vi "DoorProc_02.vi"(8 "error in":errorcluster, 11 "Cluster":T1) -> (0 "error out":errorcluster, 2 "Card Info":string, 3 "Certificate":bool=TRUE)   [LabVIEW 2011]
uses:
  Enumerator/CmdType.ctl
  DLL/Certificate_01.vi
  Interface/SockeHook/Hook_01.vi
  Variable/gSIM.vi
  Interface/SockeHook/Hook_02.vi
  Look-up/CardInfo/SPR_02.vi
  DLL/Certificate_02.vi
  Variable/gSEL.vi
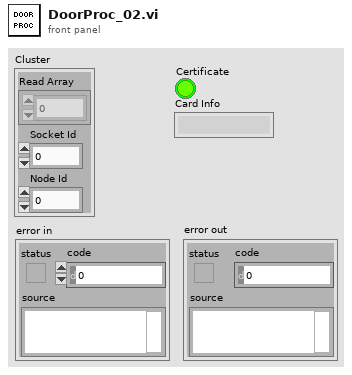
[diagram p1: front panel]
types:
  T1 = cluster{"Read Array":u8[], "Socket Id":u8, "Node Id":u8}
  T2 = enum16{"Open", "Verify", "Password", "Log", "Close"}
  T3 = enum16{"Open", "R", "W", "R->W", "W->R", "Close"}
  T4 = typedef "CmdType.ctl" = enum16{"GetEventLog", "DelTransaction", "InvalidMessage", "RelayControl", "RelayOff", "RelayOn", "VaildMessage", "EventPolling", "StoppingWaiting", "PromptKeying-in"}
  T5 = enum16{"Initial", "Insert", "Delete", "Search", "Release"}
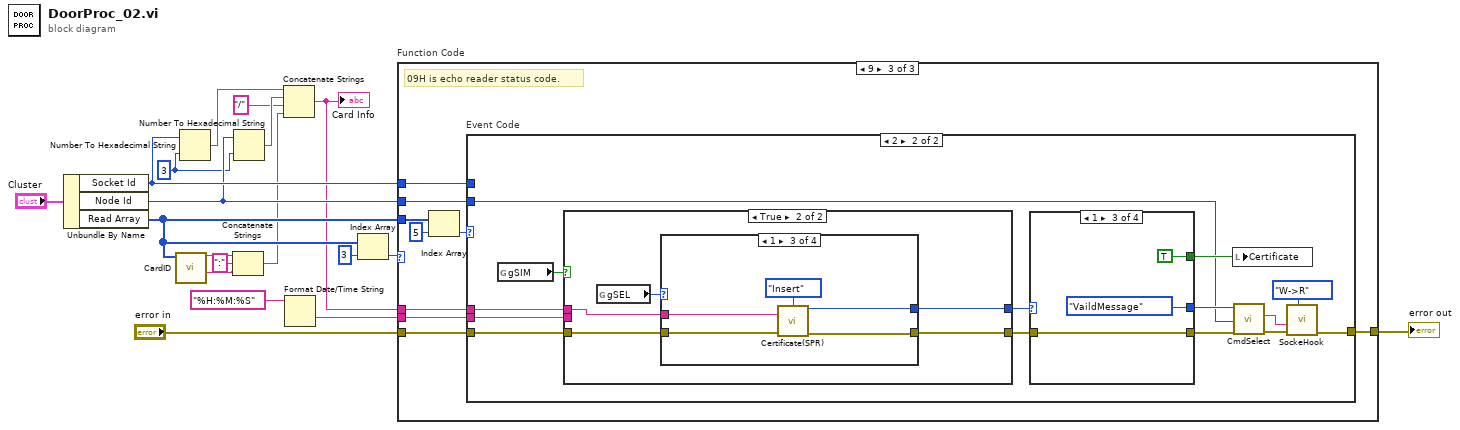
[diagram p0: block diagram]
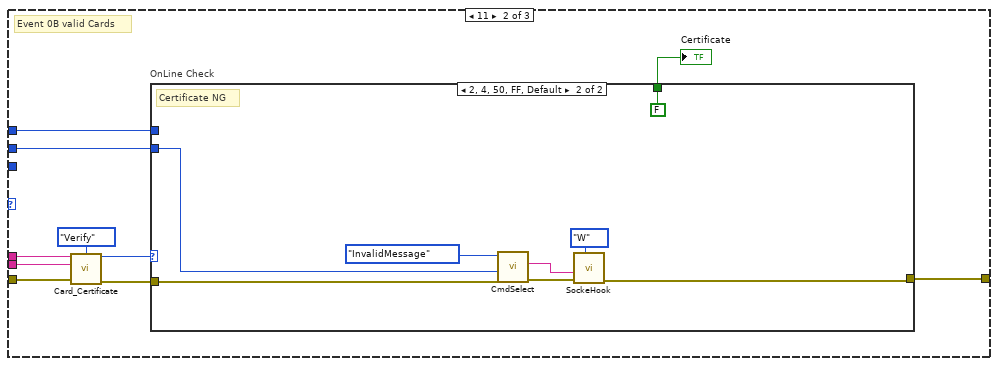
[diagram p3: hidden frame]
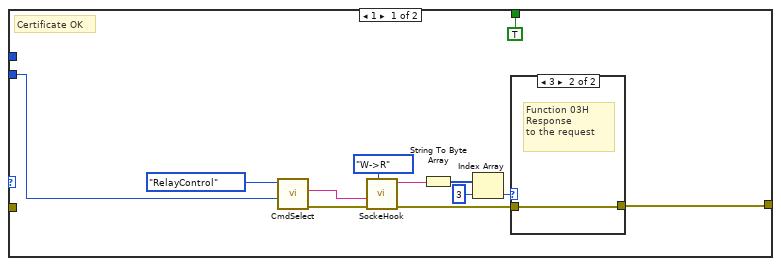
[diagram p4: hidden frame]
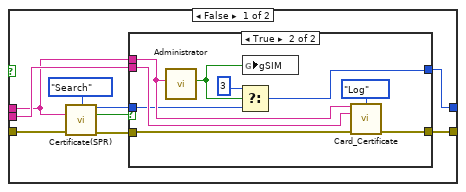
[diagram p7: hidden frame]
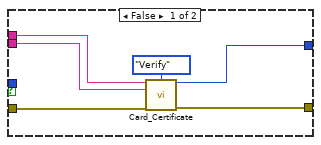
[diagram p8: hidden frame]
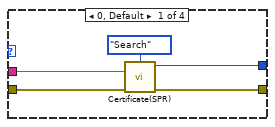
[diagram p9: hidden frame]
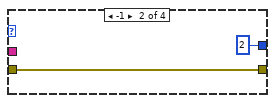
[diagram p10: hidden frame]
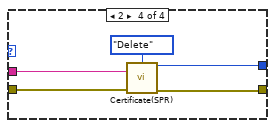
[diagram p11: hidden frame]
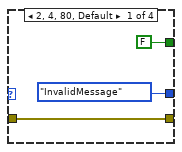
[diagram p12: hidden frame]
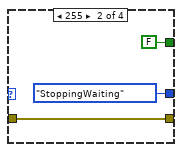
[diagram p13: hidden frame]
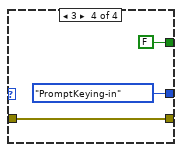
[diagram p14: hidden frame]
diagram:
  w5 = i16 3 ("width (-)")
  n1 = Unbundle By Name("Cluster") -> ("Socket Id"=w10:u8, "Node Id"=w9:u8, "Read Array"=w11:u8[])
  n2 = call "CardID.vi"("array in"=w11) -> ("Card ID"=w15:string, "Site ID"=w14:string)  [unwired: 9 in]
  n3 = Number To Hexadecimal String(1:w5, 2:w10) -> (0:w8:string)
  n4 = Concatenate Strings(w14, ":" ("string"), w15) -> (w3:string)
  n5 = Number To Hexadecimal String(1:w5, 2:w9) -> (0:w7:string)
  n6 = Concatenate Strings(w8, w7, "/" ("string"), w3) -> (w4:string)
  "Card Info" <- w4
  n7 = Format Date/Time String(time format string (%c)="%H:%M:%S") -> (date/time string=w1:string)  [unwired: 2 in]
  n8 = Index Array(array=w11, index=3) -> (element=w17:u8)
  n9 = case "Function Code" shown="9" w17 {
    tunnel: w9 -> [_ w28 w55]
    tunnel: "error in" -> [w20 w29 w58]
    tunnel: [w20 w27 w57] -> w19
    tunnel: w10 -> [_ w26 w56]
    tunnel: w11 -> [_ _ w60]
    tunnel: w1 -> [_ w24 w54]
    tunnel: w4 -> [_ w25 w53]
    frame 4, Default {
      # "04H Command Acknowledge (ACK)"
    }
    frame 11 {
      # "Event 0B valid Cards"
      n10 = call-poly "Card_Certificate.vi"("CardNumber"=w25, "DB"=T2."Verify", "Time"=w24, "error in"=w29) -> ("Certificate"=w30:u8, "error out"=w22:errorcluster)  [unwired: 10 in]
      n11 = case "OnLine Check" shown="2, 4, 50, FF, Default" w30 {
        tunnel: w28 -> [w37 w51]
        tunnel: [w38 w49] -> w27
        tunnel: w26 -> [_ _]
        tunnel: [TRUE FALSE] -> w23
        tunnel: w22 -> [_ w45]
        frame 1 {
          # "Certificate OK"
          n12 = call "CmdSelect.vi"("Node Id"=w37, "Cmd Type"=CmdType."RelayControl" ("CmdType")) -> ("error out"=w35:errorcluster, "Cmd Str"=w34:string)  [unwired: 8 in]
          n13 = call-poly "SockeHook.vi"("Mode"=T3."W->R", "error in (no error)"=w35, "data in"=w34) -> ("error out"=w33:errorcluster, "data out"=w36:string)  [unwired: 7 in]
          n14 = String To Byte Array(string=w36) -> (unsigned byte array=w41:u8[])
          n15 = Index Array(array=w41, index=3) -> (element=w39:u8)
          n16 = case shown="3" w39 {
            tunnel: w33 -> [w43 w44]
            tunnel: [w43 w44] -> w38
            frame 0, Default {
            }
            frame 3 {
              # "Function 03H\nResponse\nto the request"
            }
          }
        }
        frame 2, 4, 80, 255, Default {
          # "Certificate NG"
          n17 = call "CmdSelect.vi"("error in (no error)"=w45, "Node Id"=w51, "Cmd Type"=CmdType."InvalidMessage" ("CmdType")) -> ("error out"=w50:errorcluster, "Cmd Str"=w48:string)  [unwired: 7 in]
          n18 = call-poly "SockeHook.vi"("Mode"=T3."W", "error in (no error)"=w50, "data in"=w48) -> ("error out"=w49:errorcluster)  [unwired: 7 in, 1 out]
        }
      }
      "Certificate" <- w23
    }
    frame 9 {
      # "09H is echo reader status code."
      n19 = Index Array(array=w60, index=5) -> (element=w59:u8)
      n20 = case "Event Code" shown="2" w59 {
        tunnel: w58 -> [w62 w76]
        tunnel: [w62 w63] -> w57
        tunnel: w56 -> [_ _]
        tunnel: w55 -> [_ w64]
        tunnel: w54 -> [_ w75]
        tunnel: w53 -> [_ w66]
        frame 0, Default {
        }
        frame 2 {
          n21 = global read "gSIM.vi" "gSIM"() -> (w65:bool)
          n22 = case shown="True" w65 {
            tunnel: w76 -> [w82 w102]
            tunnel: w75 -> [w78 _]
            tunnel: [w85 w101] -> w73
            tunnel: [w84 w105] -> w72
            tunnel: w66 -> [w77 w104]
            frame False {
              n23 = call-poly "Certificate(SPR).vi"("select"=T5."Search", "key"=w77, "error in"=w82) -> ("Certificate"=w79:u8, "found"=w80:bool, "error out"=w81:errorcluster)  [unwired: 10 in]
              n24 = case shown="True" w80 {
                tunnel: [w91 w99] -> w85
                tunnel: [w90 w96] -> w84
                tunnel: w81 -> [w89 w97]
                tunnel: w79 -> [_ w93]
                tunnel: w77 -> [w87 w95]
                tunnel: w78 -> [w88 w94]
                frame False {
                  n25 = call-poly "Card_Certificate.vi"("CardNumber"=w87, "DB"=T2."Verify", "Time"=w88, "error in"=w89) -> ("Certificate"=w91:u8, "error out"=w90:errorcluster)  [unwired: 10 in]
                }
                frame True {
                  n26 = call "Administrator.vi"("string"=w95) -> ("on/off"=w98:bool)  [unwired: 10 in]
                  n27 = Select(t=u8 3 ("Certificate"), s=w98, f=w93) -> (s? t:f=w99:u8)
                  n28 = global write "gSIM.vi" "gSIM"(w98) -> ()
                  n29 = call-poly "Card_Certificate.vi"("CardNumber"=w95, "DB"=T2."Log", "Time"=w94, "error in"=w97) -> ("error out"=w96:errorcluster)  [unwired: 10 in, 1 out]
                }
              }
            }
            frame True {
              n30 = global read "gSEL.vi" "gSEL"() -> (w103:i32)
              n31 = case shown="1" w103 {
                tunnel: w102 -> [w109 w111 w116 w121]
                tunnel: [w108 w111 w115 w120] -> w105
                tunnel: [w106 u8 2 ("Certificate") w114 w119] -> w101
                tunnel: w104 -> [w107 _ w113 w118]
                frame 0, Default {
                  n32 = call-poly "Certificate(SPR).vi"("select"=T5."Search", "key"=w107, "error in"=w109) -> ("Certificate"=w106:u8, "error out"=w108:errorcluster)  [unwired: 10 in, 1 out]
                }
                frame -1 {
                }
                frame 1 {
                  n33 = call-poly "Certificate(SPR).vi"("select"=T5."Insert", "key"=w113, "error in"=w116) -> ("Certificate"=w114:u8, "error out"=w115:errorcluster)  [unwired: 10 in, 1 out]
                }
                frame 2 {
                  n34 = call-poly "Certificate(SPR).vi"("select"=T5."Delete", "key"=w118, "error in"=w121) -> ("Certificate"=w119:u8, "error out"=w120:errorcluster)  [unwired: 10 in, 1 out]
                }
              }
            }
          }
          n35 = case shown="1" w73 {
            tunnel: [CmdType."InvalidMessage" ("CmdType") CmdType."StoppingWaiting" ("CmdType") CmdType."VaildMessage" ("CmdType") CmdType."PromptKeying-in" ("CmdType")] -> w74
            tunnel: w72 -> [w124 w128 w130 w132]
            tunnel: [w124 w128 w130 w132] -> w71
            tunnel: [FALSE FALSE TRUE FALSE] -> w67
            frame 2, 4, 80, Default {
            }
            frame 255 {
            }
            frame 1 {
            }
            frame 3 {
            }
          }
          n36 = local write "Certificate"(w67) -> ()
          n37 = call "CmdSelect.vi"("error in (no error)"=w71, "Node Id"=w64, "Cmd Type"=w74) -> ("error out"=w70:errorcluster, "Cmd Str"=w69:string)  [unwired: 7 in]
          n38 = call-poly "SockeHook.vi"("Mode"=T3."W->R", "error in (no error)"=w70, "data in"=w69) -> ("error out"=w63:errorcluster)  [unwired: 7 in, 1 out]
        }
      }
    }
  }
  "error out" <- w19
